vi "GUNSC_LibUnscramble.vi"(8 "error in (no error)":errorcluster, 9 "nelems":i32, 10 "imptr":u64, 11 "rawptr":u64) -> (0 "error out":errorcluster, 2 "imptr out":u64, 3 "return value":u64)   [LabVIEW 2016]
uses:
  public/c/lib/libunsc.so
panel:
  in  "err":i32
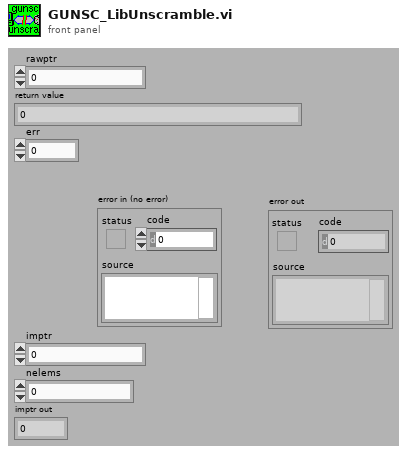
[diagram p1: front panel]
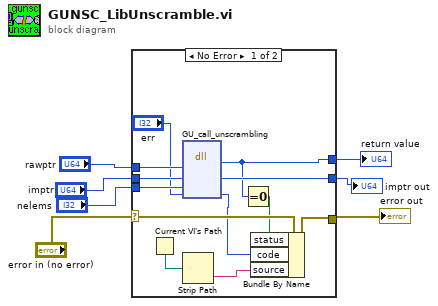
[diagram p0: block diagram]
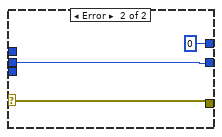
[diagram p2: hidden frame]
diagram:
  n1 = case shown="No Error" "error in (no error)" {
    selector: "error in (no error)" -> [w18 w22]
    tunnel: "rawptr" -> [w19 _]
    tunnel: [w10 0] -> w6
    tunnel: [w14 w22] -> w4
    tunnel: "imptr" -> [w13 w20]
    tunnel: "nelems" -> [w12 _]
    tunnel: [w11 w20] -> w1
    frame No Error {
      n2 = Current VI's Path() -> (path=w16:path)
      n3 = dll-call lib="home/simager/panview/PAN/Modules/GUNSC/public/c/lib/libunsc.so" fn="GU_call_unscrambling"("rawptr"=w19, "imptr"=w13, "nelems"=w12, "err"="err") -> ("return type"=w10:u64, "imptr"=w11:u64, "err"=w8:i32)  [unwired: 5 in, 2 out]
      n4 = Strip Path(path=w16) -> (name=w15:string)  [unwired: 1 out]
      n5 = Equal To 0?(x=w10) -> (x = 0?=w17:bool)
      n6 = Bundle By Name(cluster=w18, "status"=w17, "code"=w8, "source"=w15) -> (w14:errorcluster)
    }
    frame Error {
    }
  }
  "return value" <- w6
  "error out" <- w4
  "imptr out" <- w1
